vi "Basic Usage.vi"() -> ()   [LabVIEW 2017]
uses:
  SubVIs/Command Queue Data.ctl
  Futures/Promise/Promise.lvclass
  Futures/Future/Future.lvclass
panel:
  out "Result":dbl
  out "result error":errorcluster
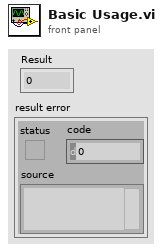
[diagram p1: front panel]
types:
  T1 = typedef "Command Queue Data.ctl" = cluster{"Promise":refnum<class "Promise.lvclass">, "notifier":refnum<notifier>}
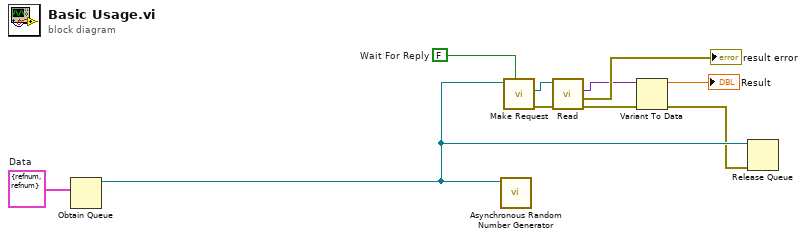
[diagram p0: block diagram]
diagram:
  w8 = FALSE  # Wait For Reply
  w10 = T1 {"Promise"=refnum, "notifier"=refnum}  # Data
  n1 = Obtain Queue(element data type=w10) -> (queue out=w9:refnum<queue>)  [unwired: 4 in, 2 out]
  n2 = call "Asynchronous Random Number Generator.vi"("Queue in"=w9) -> ()  [unwired: 11 in]
  n3 = call "Make Request.vi"("Wait For Reply"=w8, "Worker Queue"=w9) -> ("error out"=w7:errorcluster, "Future"=w6:refnum<class "Future.lvclass">)  [unwired: 8 in]
  n4 = call "Read.vi"("error in (no error)"=w7, "Future in"=w6) -> ("error out"=w5:errorcluster, "result error"=→"result error":errorcluster, "Result value"=w2:variant)  [unwired: 6 in, 1 out]
  n5 = Variant To Data(error in=w5, Variant=w2) -> (data=→"Result":dbl, error out=w4:errorcluster)  [unwired: 1 in]
  n6 = Release Queue(queue=w9, error in (no error)=w4) -> ()  [unwired: 1 in, 3 out]
